vi "SCT Merge Attributes.vi"(10 "New Attribs":T4, 11 "Variable In":T1) -> (2 "Ambiguous?":bool, 3 "Variable out":T1)   [LabVIEW 2016]
uses:
  <resource>/dialog/variable/SCT Attribute Changes.ctl
  <resource>/dialog/variable/SCT Variable.ctl
  <vilib>/variable/Type Descriptor.ctl
  <vilib>/variable/Attribs.ctl
  <vilib>/variable/NI_Variable.lvlib
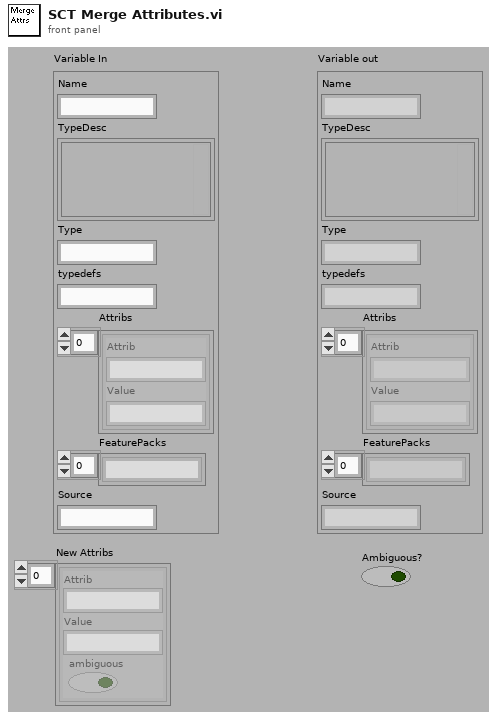
[diagram p1: front panel]
types:
  T1 = typedef "SCT Variable.ctl" = cluster{"Name":string, "TypeDesc":T2, "Type":string, "typedefs":string, "Attribs":T3, "FeaturePacks":string[], "Source":string}
  T2 = typedef "NI_Variable.lvlib/Type Descriptor.ctl" = cluster{"Variant":variant}
  T3 = typedef "NI_Variable.lvlib/Attribs.ctl" = cluster{"Attrib":string, "Value":string}[]
  T4 = typedef "SCT Attribute Changes.ctl" = cluster{"Attrib":string, "Value":string, "ambiguous":bool}[]
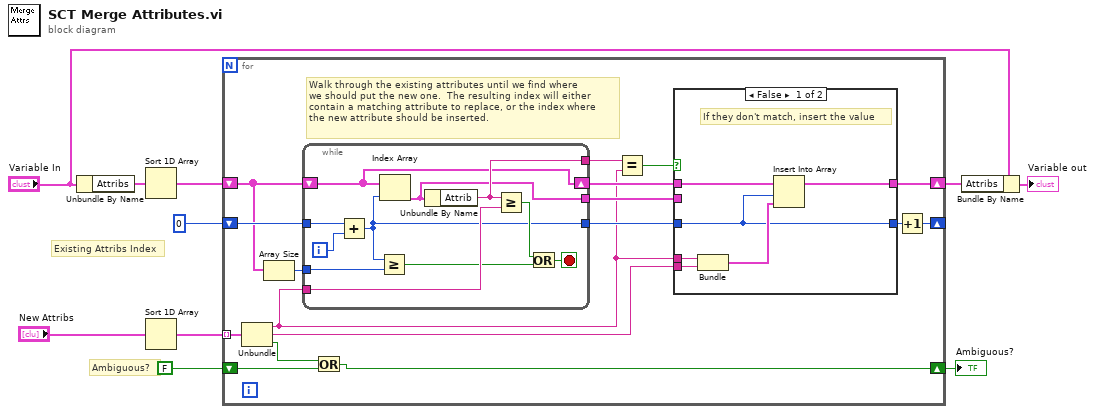
[diagram p0: block diagram]
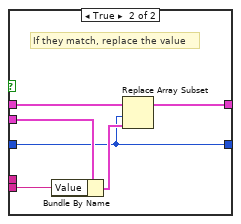
[diagram p2: hidden frame]
diagram:
  # "Existing Attribs Index"
  # "Ambiguous?"
  n1 = Unbundle By Name("Variable In") -> ("Attribs"=w3:T3)
  n2 = Sort 1D Array(array=w3) -> (sorted array=w9:T3)
  n3 = Sort 1D Array(array="New Attribs") -> (sorted array=w8:T4)
  n4 = for {
    shift-right: [w23] -> w1
    shift-left: FALSE -> [w25]
    shift-right: [w11] -> _
    shift-left: 0 -> [w27]
    shift-right: [w13] -> w5
    shift-left: w9 -> [w22]
    tunnel: w8 -> [w26] mode=indexing
    # "Walk through the existing attributes until we find where\nwe should put the new one.  The resulting index will either\ncontain a matching attribute to replace, or the index where\nthe new attribute should be inserted."
    n5 = Unbundle(w26) -> ("Attrib"=w14:string, "Value"=w16:string, "ambiguous"=w24:bool)
    n6 = Array Size(array=w22) -> (size(s)=w21:i32)
    n7 = while {
      tunnel: w27 -> [w49]
      tunnel: w14 -> [w48]
      tunnel: w21 -> [w47]
      tunnel: [w43] -> w15
      tunnel: [w42] -> w20
      shift-right: [w41] -> w18
      shift-left: w22 -> [w41]
      tunnel: [w40] -> w17
      i -> [w50]
      stop <- w44 stop-if-true
      n8 = Add(x=w49, y=w50) -> (x+y=w43:i32)
      n9 = Greater Or Equal?(x=w43, y=w47) -> (x >= y?=w45:bool)
      n10 = Index Array(array=w41, index=w43) -> (element=w40:cluster{"Attrib":string, "Value":string})
      n11 = Unbundle By Name(w40) -> ("Attrib"=w42:string)
      n12 = Greater Or Equal?(x=w42, y=w48) -> (x >= y?=w46:bool)
      n13 = Or(x=w46, y=w45) -> (x .or. y?=w44:bool)
    }
    n14 = Or(x=w24, y=w25) -> (x .or. y?=w23:bool)
    n15 = Equal?(x=w20, y=w14) -> (x = y?=w19:bool)
    n16 = case shown="False" w19 {
      tunnel: w18 -> [w32 w37]
      tunnel: w17 -> [_ w39]
      tunnel: w16 -> [w31 w38]
      tunnel: w15 -> [w28 w34]
      tunnel: [w33 w35] -> w13
      tunnel: w14 -> [w30 _]
      tunnel: [w28 w34] -> w12
      frame False {
        # "If they don't match, insert the value"
        n17 = Bundle("Attrib"=w30, "Value"=w31) -> (w29:cluster{"Attrib":string, "Value":string})  [unwired: 1 in]
        n18 = Insert Into Array(array=w32, index=w28, new element=w29) -> (w33:T3)
      }
      frame True {
        # "If they match, replace the value"
        n19 = Bundle By Name(cluster=w39, "Value"=w38) -> (w36:cluster{"Attrib":string, "Value":string})
        n20 = Replace Array Subset(array=w37, new element=w36, index=w34) -> (w35:T3)
      }
    }
    n21 = Increment(x=w12) -> (x+1=w11:i32)
  }
  "Ambiguous?" <- w1
  n22 = Bundle By Name(cluster="Variable In", "Attribs"=w5) -> (→"Variable out":T1)
